vi "UpdateInventorySabritas.vi"(8 "error in (no error)":errorcluster, 11 "Sabritas Actor in":refnum<class "Sabritas Actor.lvclass">) -> (0 "error out":errorcluster, 3 "Sabritas Actor out":refnum<class "Sabritas Actor.lvclass">)   [LabVIEW 2020, in "Sabritas Actor.lvlib" / "Sabritas Actor.lvclass"]
uses:
  Sabritas Actor.lvclass
  Sabritas Actor.lvclass/Sabritas Actor.ctl
  <vilib>/Utility/config.llb/Read Key (Double).vi
  <vilib>/Utility/config.llb/Read Key (String).vi
  <vilib>/Utility/config.llb/NI_LVConfig.lvlib
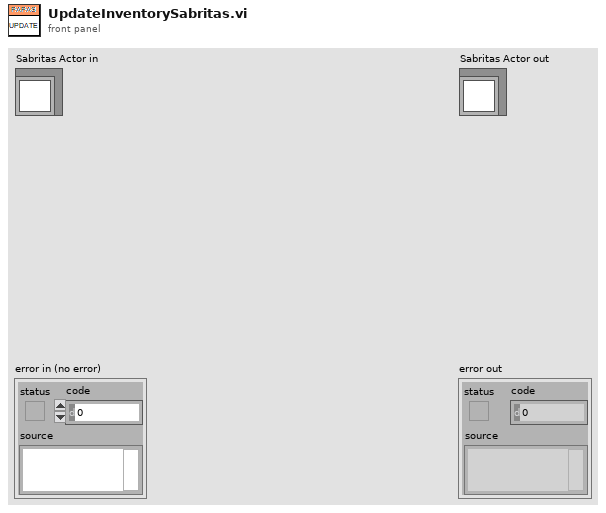
[diagram p1: front panel]
types:
  T1 = typedef "NI_LVConfig.lvlib/Config Data RefNum.ctl" = refnum<k1>
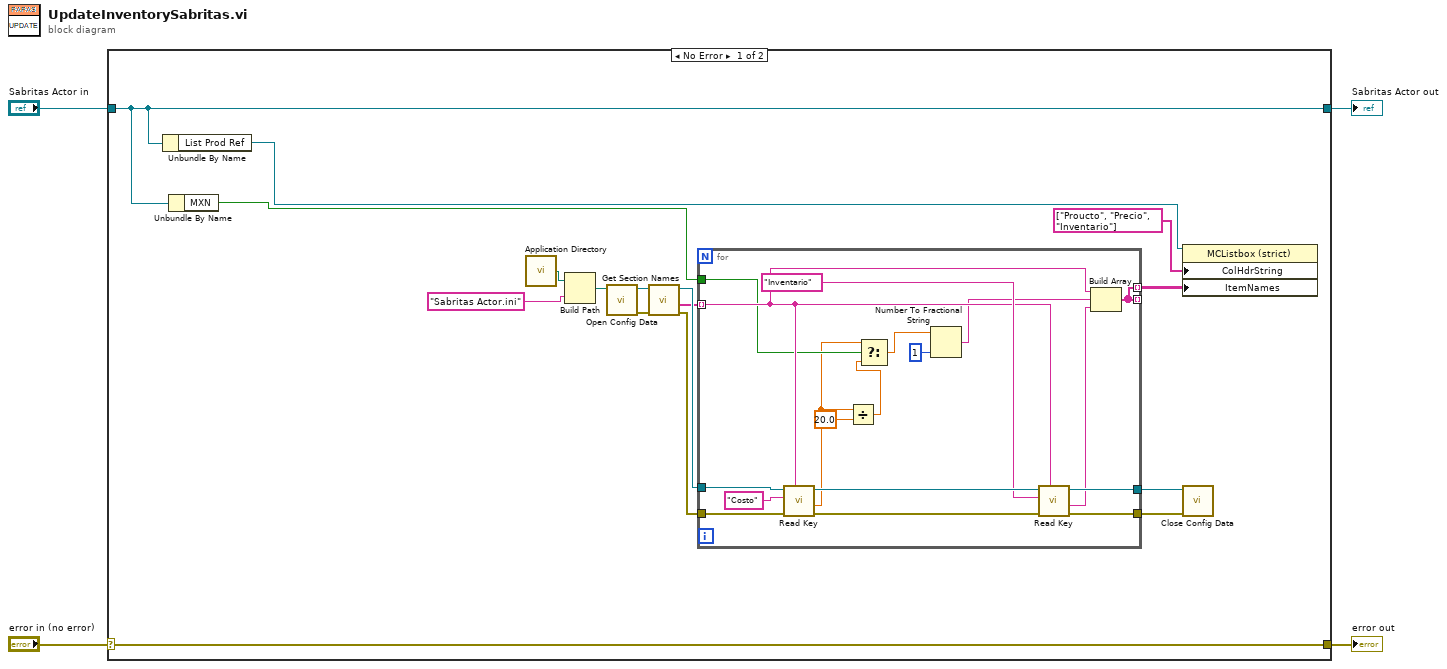
[diagram p0: block diagram]
diagram:
  n1 = case shown="No Error" "error in (no error)" {
    selector: "error in (no error)" -> [w20 w40]
    tunnel: [w20 w40] -> w3
    tunnel: [w5 w39] -> w1
    tunnel: "Sabritas Actor in" -> [w5 w39]
    frame No Error {
      n2 = Unbundle By Name(w5) -> ("List Prod Ref"=w8:refnum<vi>)
      n3 = Unbundle By Name(w5) -> ("MXN"=w13:bool)
      n4 = call <vilib>:"Application Directory.vi"() -> ("Application Directory"=w18:path)
      n5 = Build Path(base path=w18, name or relative path="Sabritas Actor.ini") -> (appended path=w17:path)
      n6 = call <vilib>:"Open Config Data.vi"("configuration file path"=w17) -> ("error out"=w16:errorcluster, "refnum"=w11:T1)  [unwired: 8 in, 1 out]
      n7 = call <vilib>:"Get Section Names.vi"("error in (no error)"=w16, "refnum"=w11) -> ("error out"=w12:errorcluster, "section names"=w9:string[], "refnum out"=w10:T1)  [unwired: 7 in]
      n8 = for {
        tunnel: w10 -> [w38]
        tunnel: w12 -> [w37]
        tunnel: [w33] -> w15
        tunnel: [w34] -> w14
        tunnel: w13 -> [w25]
        tunnel: w9 -> [w30] mode=indexing
        tunnel: [w28] -> _ mode=indexing
        tunnel: [w28] -> w7 mode=indexing
        n9 = call-poly <vilib>:"Read Key.vi"("section"=w30, "error in (no error)"=w37, "key"="Costo", "refnum"=w38) -> ("error out"=w35:errorcluster, "value"=w23:dbl, "refnum out"=w36:T1)  [unwired: 4 in, 1 out]
        n10 = Divide(x=w23, y=20.0) -> (x/y=w21:dbl)
        n11 = Select(t=w23, s=w25, f=w21) -> (s? t:f=w24:dbl)
        n12 = Number To Fractional String(number=w24, precision (6)=i16 1) -> (F-format string=w26:string)  [unwired: 2 in]
        n13 = call-poly <vilib>:"Read Key.vi"("section"=w30, "error in (no error)"=w35, "key"="Inventario", "refnum"=w36) -> ("error out"=w33:errorcluster, "value"=w29:string, "refnum out"=w34:T1)  [unwired: 4 in, 1 out]
        n14 = Build Array(w30, w26, w29) -> (w28:string[])
      }
      n15 = property class="MCListbox (strict)"(reference=w8, "ColHdrString"=string[] ["Proucto", "Precio", "Inventario"] ("Column Header Strings[]"), "ItemNames"=w7) -> ()  [unwired: 1 in, 2 out]
      n16 = call <vilib>:"Close Config Data.vi"("error in (no error)"=w15, "refnum"=w14) -> ()  [unwired: 8 in, 2 out]
    }
    frame Error {
    }
  }
  "error out" <- w3
  "Sabritas Actor out" <- w1
